vi "M10 TV.vi"(11 "NXT/EV3":T1) -> (3 "EV3 out":T1)   [LabVIEW 2016]
uses:
  <vilib>/NXT/Subs/LVHSConnector.ctl
  <vilib>/NXT/LegoClasses/BrickReference/BrickReference.lvclass
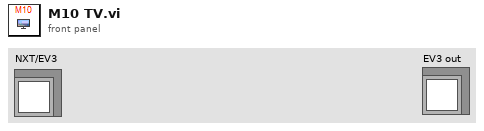
[diagram p1: front panel]
types:
  T1 = typedef "LVHSConnector.ctl" = refnum<class "BrickReference.lvclass">
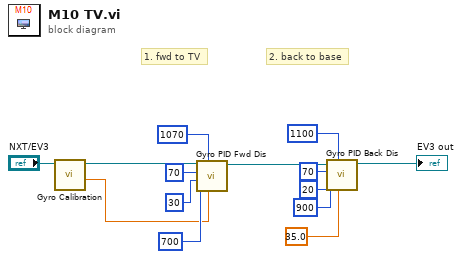
[diagram p0: block diagram]
diagram:
  # "2. back to base"
  # "1. fwd to TV"
  n1 = call "Gyro Calibration.vi"("NXT/EV3"="NXT/EV3") -> ("Degrees"=w4:sgl, "NXT/EV3"=w2:T1)  [unwired: 6 in, 1 out]
  n2 = call "Gyro PID Fwd Dis.vi"("Target angle"=w4, "Threshold to stop"=1070, "Threshold to slow"=700, "Min. speed"=30, "Max. speed"=70, "EV3 in"=w2) -> ("EV3 out"=w9:T1)  [unwired: 5 in]
  n3 = call "Gyro PID Back Dis.vi"("Target angle"=sgl 35.0, "Threshold to stop"=1100, "Threshold to slow"=900, "Min. speed"=20, "Max. speed"=70, "EV3 in"=w9) -> ("EV3 out"=→"EV3 out":T1)  [unwired: 5 in]
